vi "Main.vi"() -> ()   [LabVIEW 2014]
uses:
  <vilib>/lvrevbrd/DiffVIs.lvlib
panel:
  out "Application:Command Line Arguments":string[](array[string])
  out "path2":path
  out "path1":path
  out "caption 2":string
  out "output directory":path
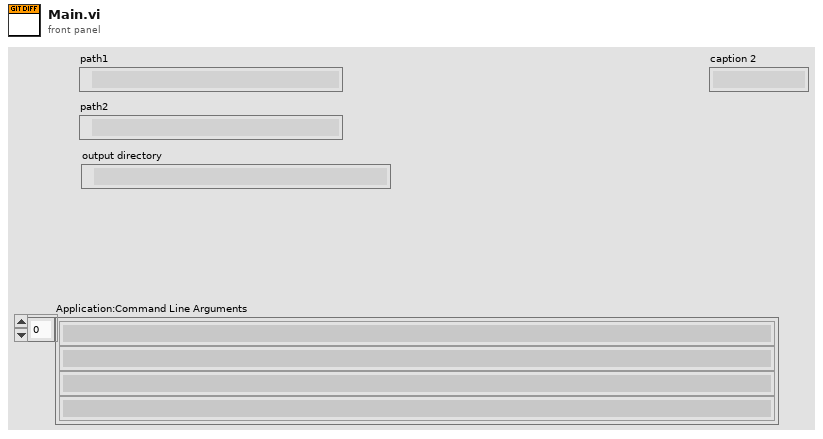
[diagram p1: front panel]
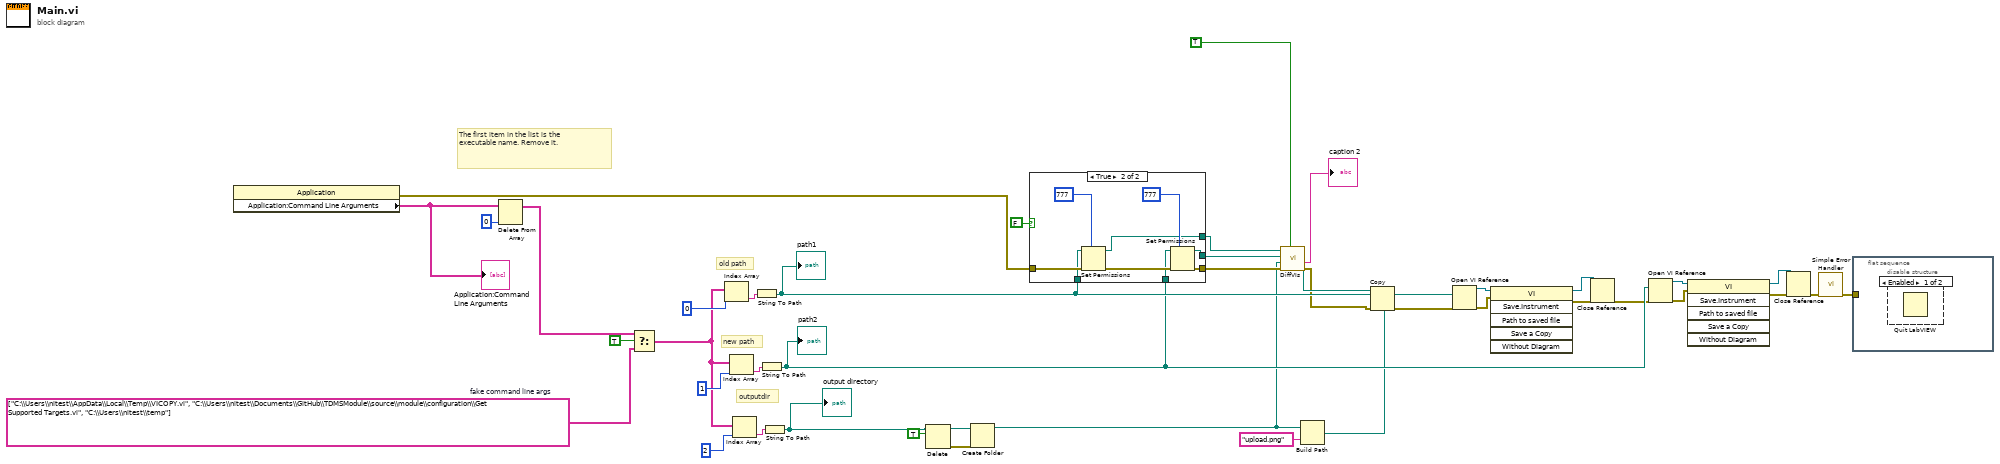
[diagram p0: block diagram]
diagram:
  w28 = string[] ["C:\\Users\\nitest\\AppData\\Local\\Temp\\VICOPY.vi", "C:\\Users\\nitest\\Documents\\GitHub\\TDMSModule\\source\\module\\configuration\\Get Supported Targets.vi", "C:\\Users\\nitest\\temp"]  # fake command line args
  # "outputdir"
  # "new path"
  # "old path"
  # "The first item in the list is the executable name. Remove it."
  n1 = property class="Application"() -> (error out=w37:errorcluster, "Application:Command Line Arguments"=w39:string[])  [unwired: 2 in, 1 out]
  "Application:Command Line Arguments" <- w39
  n2 = Delete From Array(array=w39, index=0 ("length")) -> (array with subset deleted=w27:string[])  [unwired: 1 in, 1 out]
  n3 = Select(t=w27, s=TRUE, f=w28) -> (s? t:f=w26:string[])
  n4 = Index Array(array=w26, index=0) -> (element=w35:string)
  n5 = Index Array(array=w26, index=1) -> (element=w34:string)
  n6 = Index Array(array=w26, index=2) -> (element=w31:string)
  n7 = String To Path(string=w35) -> (path=w19:path)
  "path1" <- w19
  n8 = String To Path(string=w34) -> (path=w8:path)
  "path2" <- w8
  n9 = String To Path(string=w31) -> (path=w23:path)
  "output directory" <- w23
  n10 = Delete(path (use dialog)=w23, entire hierarchy (F)=TRUE) -> (deleted path=w20:path, error out=w21:errorcluster)  [unwired: 3 in, 1 out]
  n11 = Create Folder(path (use dialog)=w20, error in=w21) -> (created path=w4:path)  [unwired: 1 in, 2 out]
  n12 = case shown="True" FALSE {
    tunnel: [w43 w51] -> w41
    tunnel: w37 -> [w43 w50]
    tunnel: w8 -> [w44 w49]
    tunnel: w19 -> [w45 w48]
    tunnel: [w45 w47] -> w30
    tunnel: [w44 w46] -> w29
    frame False {
      # "delete this BS"
    }
    frame True {
      n13 = Set Permissions(7:i16 777 ("permissions"), 8:w50, 11:w48) -> (0:w52:errorcluster, 3:w47:path)  [unwired: 2 in]
      n14 = Set Permissions(7:i16 777 ("permissions"), 8:w52, 11:w49) -> (0:w51:errorcluster, 3:w46:path)  [unwired: 2 in]
    }
  }
  n15 = call <vilib>:"DiffVIs.vi"("Take ScrShots All In"=TRUE, "error in"=w41, "Picture Save Location"=w4, "VI Path 2"=w29, "VI Path 1"=w30) -> ("error out"=w1:errorcluster, "caption"=→"caption 2":string, "diff file"=w6:path)  [unwired: 2 in, 2 out]
  n16 = Build Path(base path=w4, name or relative path="upload.png") -> (appended path=w5:path)
  n17 = Copy(8:w1, 10:w5, 11:w6) -> (0:w2:errorcluster)  [unwired: 2 in, 2 out]
  n18 = Open VI Reference(vi path=w19, error in (no error)=w2) -> (vi reference=w18:refnum<vi>, error out=w17:errorcluster)  [unwired: 4 in]
  n19 = invoke class="VI" method="Save.Instrument"(reference=w18, error in=w17) -> (reference out=w15:refnum<vi>, error out=w16:errorcluster)  [unwired: 4 in, 4 out]
  n20 = Close Reference(reference=w15, error in (no error)=w16) -> (error out=w7:errorcluster)
  n21 = Open VI Reference(vi path=w8, error in (no error)=w7) -> (vi reference=w10:refnum<vi>, error out=w11:errorcluster)  [unwired: 4 in]
  n22 = invoke class="VI" method="Save.Instrument"(reference=w10, error in=w11) -> (reference out=w13:refnum<vi>, error out=w12:errorcluster)  [unwired: 4 in, 4 out]
  n23 = Close Reference(reference=w13, error in (no error)=w12) -> (error out=w9:errorcluster)
  n24 = call <vilib>:"Simple Error Handler.vi"("error in (no error)"=w9) -> ("error out"=w14:errorcluster)  [unwired: 4 in, 4 out]
  n25 = flat-sequence {
    tunnel: w14 -> [_]
    frame #0 {
      n26 = disable-structure shown="Enabled" {
        frame Enabled {
          n27 = Quit LabVIEW() -> ()  [unwired: 1 in]
        }
        frame Disabled {
        }
      }
    }
  }
